vi "Send and Receive Message.vi"(4 "timeout (ms) [100]":i32=100, 6 "Wait for response [T]":bool=TRUE, 8 "error in (no error)":errorcluster, 9 "Data":variant, 10 "Command":string, 11 "RemoteControl in":refnum<class "RemoteControl.lvclass">) -> (0 "error out":errorcluster, 1 "Data out":variant, 2 "Command out":string, 3 "RemoteControl out":refnum<class "RemoteControl.lvclass">)   [LabVIEW 2020, in "RemoteControl.lvclass"]
uses:
  RemoteControl.lvclass
  <userlib>/_OpenG.lib/numeric/numeric.llb/Random Number Within Range - I32__ogtk.vi
  <vilib>/Utility/error.llb/Error Cluster From Error Code.vi
  <vilib>/ErrorRing/Error Ring.xnode
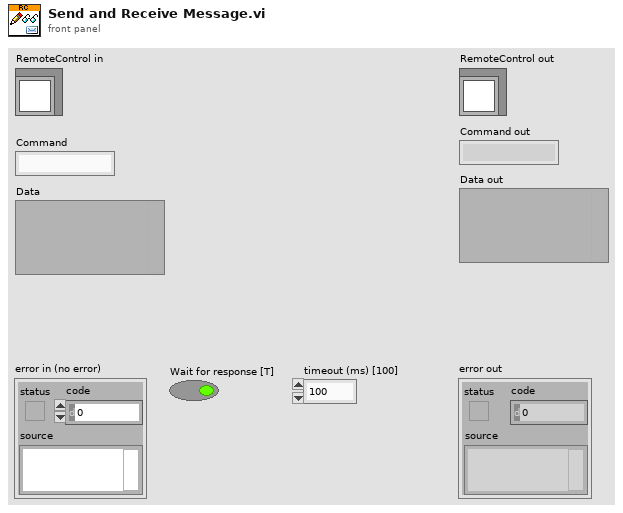
[diagram p1: front panel]
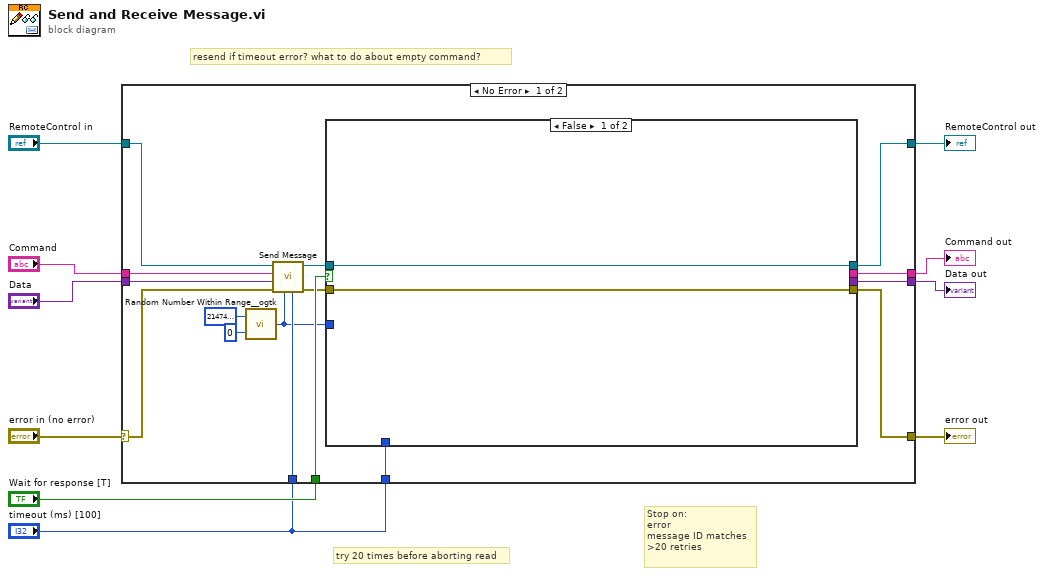
[diagram p0: block diagram]
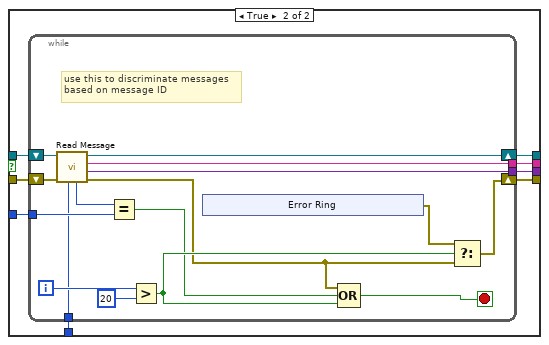
[diagram p2: hidden frame]
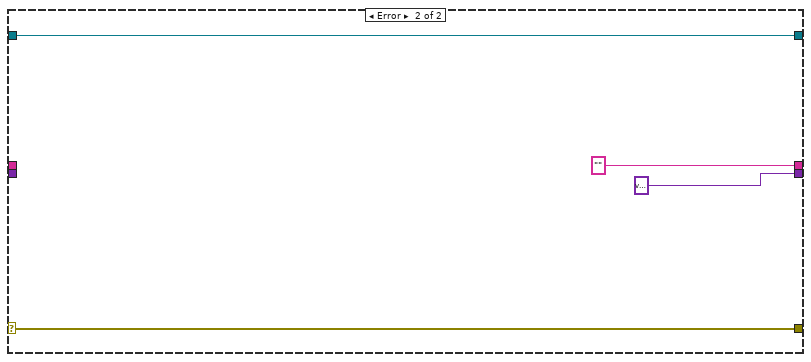
[diagram p3: hidden frame]
diagram:
  # "Stop on:\nerror\nmessage ID matches\n>20 retries"
  # "resend if timeout error? what to do about empty command?"
  # "try 20 times before aborting read"
  n1 = case shown="No Error" "error in (no error)" {
    selector: "error in (no error)" -> [w21 w60]
    tunnel: [w12 w60] -> w9
    tunnel: [w19 w59] -> w7
    tunnel: "RemoteControl in" -> [w22 w59]
    tunnel: "Wait for response [T]" -> [w26 _]
    tunnel: "timeout (ms) [100]" -> [w25 _]
    tunnel: "timeout (ms) [100]" -> [w20 _]
    tunnel: "Command" -> [w11 _]
    tunnel: "Data" -> [w18 _]
    tunnel: [w17 "" ("Command")] -> w4
    tunnel: [w16 variant ("Data")] -> w3
    frame No Error {
      n2 = call-poly <userlib>:"Random Number Within Range__ogtk.vi"("High"=2147483647, "Low"=0) -> ("Random Number"=w13:i32)  [unwired: 3 in]
      n3 = call-dynamic "Send Message.vi"("timeout in ms (100)"=w20, "Message ID"=w13, "error in (no error)"=w21, "Data"=w18, "Command"=w11, "RemoteControl in"=w22) -> ("error out"=w23:errorcluster, "RemoteControl out"=w24:refnum<class "RemoteControl.lvclass">)  [unwired: 4 in]
      n4 = case shown="False" w26 {
        tunnel: w24 -> [w27 w36]
        tunnel: [w27 w35] -> w19
        tunnel: [_ w34] -> w17
        tunnel: [_ w33] -> w16
        tunnel: [w28 w32] -> w12
        tunnel: w23 -> [w28 w31]
        tunnel: w25 -> [_ w30]
        tunnel: w13 -> [_ w29]
        frame False {
        }
        frame True {
          n5 = while {
            tunnel: [w44] -> w34
            tunnel: [w50] -> w33
            tunnel: w30 -> [w43]
            shift-right: [w51] -> w35
            shift-left: w36 -> [w52]
            shift-right: [w40] -> w32
            shift-left: w31 -> [w49]
            tunnel: w29 -> [w45]
            i -> [w47]
            stop <- w46 stop-if-true
            # "use this to discriminate messages\nbased on message ID"
            n6 = call-dynamic "Read Message.vi"("timeout in ms (100)"=w43, "error in (no error)"=w49, "RemoteControl in"=w52) -> ("error out"=w38:errorcluster, "Data"=w50:variant, "Command"=w44:string, "RemoteControl out"=w51:refnum<class "RemoteControl.lvclass">, "Message ID"=w42:i32)  [unwired: 4 in]
            n7 = Equal?(x=w42, y=w45) -> (x = y?=w37:bool)
            n8 = Greater?(x=w47, y=20) -> (0:w41:bool)
            n9 = xnode "Error Ring"() -> ("error out"=w39:errorcluster)
            n10 = Compound Arithmetic op=OR(w38, w37, w41) -> (w46:bool)
            n11 = Select(t=w39, s=w41, f=w38) -> (s? t:f=w40:errorcluster)
          }
        }
      }
    }
    frame Error {
    }
  }
  "error out" <- w9
  "RemoteControl out" <- w7
  "Command out" <- w4
  "Data out" <- w3
